vi "InitializeLED.vi"(8 "error in (no error)":errorcluster) -> (0 "error out":errorcluster)   [LabVIEW 2015]
uses:
  PacDriveSDK/C#/bin/Debug/PacDrive32.dll
panel:
  out "#boards":i32
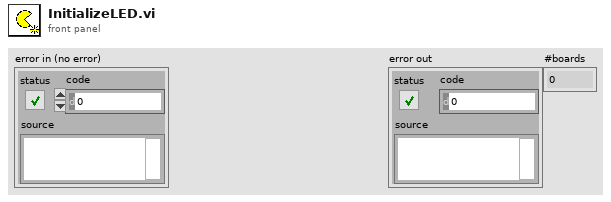
[diagram p1: front panel]
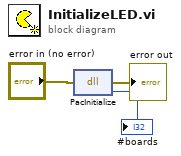
[diagram p0: block diagram]
diagram:
  n1 = dll-call lib="C:/Users/Team4153/Documents/GitHub/2016_competition/2016 Dashboard Project/TestLights Folder/PacDriveSDK/C#/bin/Debug/PacDrive32.dll" fn="PacInitialize"(error in="error in (no error)") -> (error out=→"error out":errorcluster, "return type"=→"#boards":i32)  [unwired: 2 in, 1 out]
